vi "FGV user laser 1 wavelength.vi"(7 "FGV Actions":enum16{"Get", "Set user wavelength"}(ring), 8 "error in (no error)":errorcluster, 11 "Laser wavelength IN":dbl) -> (0 "error out":errorcluster, 3 "Laser wavelength OUT":dbl)   [LabVIEW 2017]
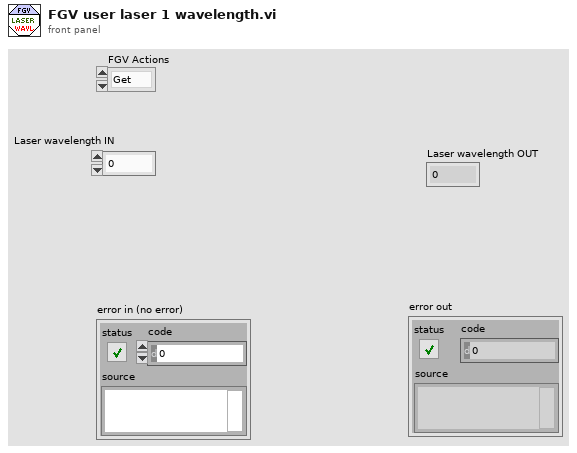
[diagram p1: front panel]
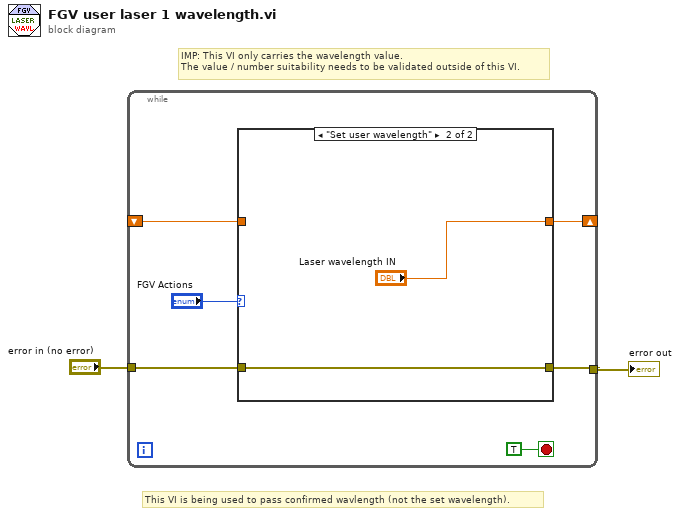
[diagram p0: block diagram]
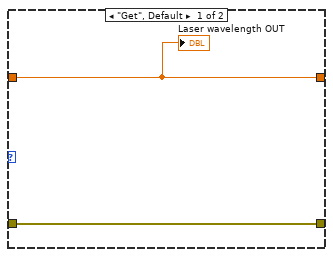
[diagram p2: hidden frame]
diagram:
  # "This VI is being used to pass confirmed wavlength (not the set wavelength)."
  # "IMP: This VI only carries the wavelength value.\nThe value / number suitability needs to be validated outside of this VI."
  n1 = while {
    shift-right: [w6] -> _
    shift-left: _ -> [w5]
    tunnel: "error in (no error)" -> [w4]
    tunnel: [w3] -> w1
    stop <- TRUE stop-if-true
    n2 = case shown="\"Set user wavelength\"" "FGV Actions" {
      tunnel: [w10 "Laser wavelength IN"] -> w6
      tunnel: w5 -> [w10 _]
      tunnel: w4 -> [w9 w12]
      tunnel: [w9 w12] -> w3
      frame "Get", Default {
        "Laser wavelength OUT" <- w10
      }
      frame "Set user wavelength" {
      }
    }
  }
  "error out" <- w1
